vi "XIPIN_Utility_idelayctrl_1_0.vi"   [LabVIEW 2017]
doc: "util_idelay_ctrl_v1_0\n------------------------------------\n<b>Need License</b> : No"
uses:
  <vilib>/rvi/XilinxIP/XIPIN_XNode/niFpgaXIPIN.xnode
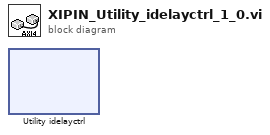
[diagram p0: block diagram]
diagram:
  n1 = xnode ("Utility idelayctrl")() -> ()
